vi "serpOpen.vi_(6-port_edit).vi"() -> ()   [LabVIEW 2010]
panel:
  in  "out driver names":string[](array[string])=[".aOut", ".bOut", ".cOut", ".dOut", ".eOut", ".fOut"]
  in  "input driver names":string[](array[string])=[".aIn", ".bIn", ".cIn", ".dIn", ".eIn", ".fIn"]
  out "driver opened":bool[](array[boolean])
  # "Replace in sersup.llb if serial errors encountered\nRemove (6- port edit) from name"
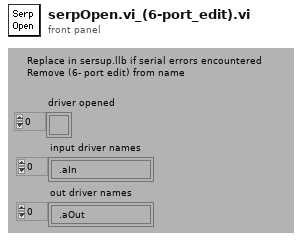
[diagram p1: front panel]
diagram:
